vi "Graph ERD Read List.vi"(0 "GEA2 Reference In":refnum<k24>, 5 "GEA Inputs":T10={"Source"=240, "Destination"=35} {"Destination" format="%.0x"; "Source" format="%.0x"}, 7 "ERD_Data_Bundled_In":T1, 9 "ERD Graph Cntrl":T11={"ERD 3"={"ERD #"=0, "Data Type"=enum."uint16_t", "Scaler"=1}, "ERD 2"={"ERD #"=0, "Data Type"=enum."uint16_t", "Scaler"=1}, "ERD 1"={"ERD #"=0, "Data Type"=enum."uint16_t", "Scaler"=1}} {"ERD 1"."Scaler" min=1; "ERD 1"."ERD #" format="%.0x"; "ERD 2"."Scaler" min=1; "ERD 2"."ERD #" format="%.0x"; "ERD 3"."Scaler" min=1; "ERD 3"."ERD #" format="%.0x"}, 11 "Error In":errorcluster) -> (4 "GEA2 Reference Out":refnum<k24>, 6 "ERD Graph  Ind":T9, 8 "ERD_Data_Bundled_Out":T1, 15 "Error Out":errorcluster)   [LabVIEW 2014]
uses:
  Common/LabVIEW GEA2 Toolkit/LabVIEW_GEA2_Toolkit.lvlibp/type defs/ERD Read Data In.ctl
  Common/LabVIEW GEA2 Toolkit/LabVIEW_GEA2_Toolkit.lvlibp
  Common/LabVIEW GEA2 Toolkit/LabVIEW_GEA2_Toolkit.lvlibp/type defs/Data Type.ctl
  type defs/ERD_Graph.ctl
  type defs/ERD_Graph_All.ctl
  C:/Automation/DLLs/PC Dot Net/GeaCommunication.dll
  Common/LabVIEW GEA2 Toolkit/LabVIEW_GEA2_Toolkit.lvlibp/type defs/Source_Destination.ctl
  type defs/ATC_Data.ctl
  type defs/Redundant.ctl
  type defs/Version.ctl
  type defs/Algorithms.ctl
  type defs/ERD_Always_Show.ctl
  type defs/ERD_Data_Bundled.ctl
  type defs/Fault_Table_Info.ctl
  type defs/Cycle_Diag.ctl
panel:
  # "Wet Load Size"
  # "Dry Load Size"
  # "OOB"
  # "Software Version"
  # "Critical Version"
  # "Non-Critical"
  # "XML Crit Ver"
  # "XML Non-Crit"
  # "Daily Build"
  # "Wet Load Size"
  # "Dry Load Size"
  # "OOB"
  # "Software Version"
  # "Critical Version"
  # "Non-Critical"
  # "XML Crit Ver"
  # "XML Non-Crit"
  # "Daily Build"
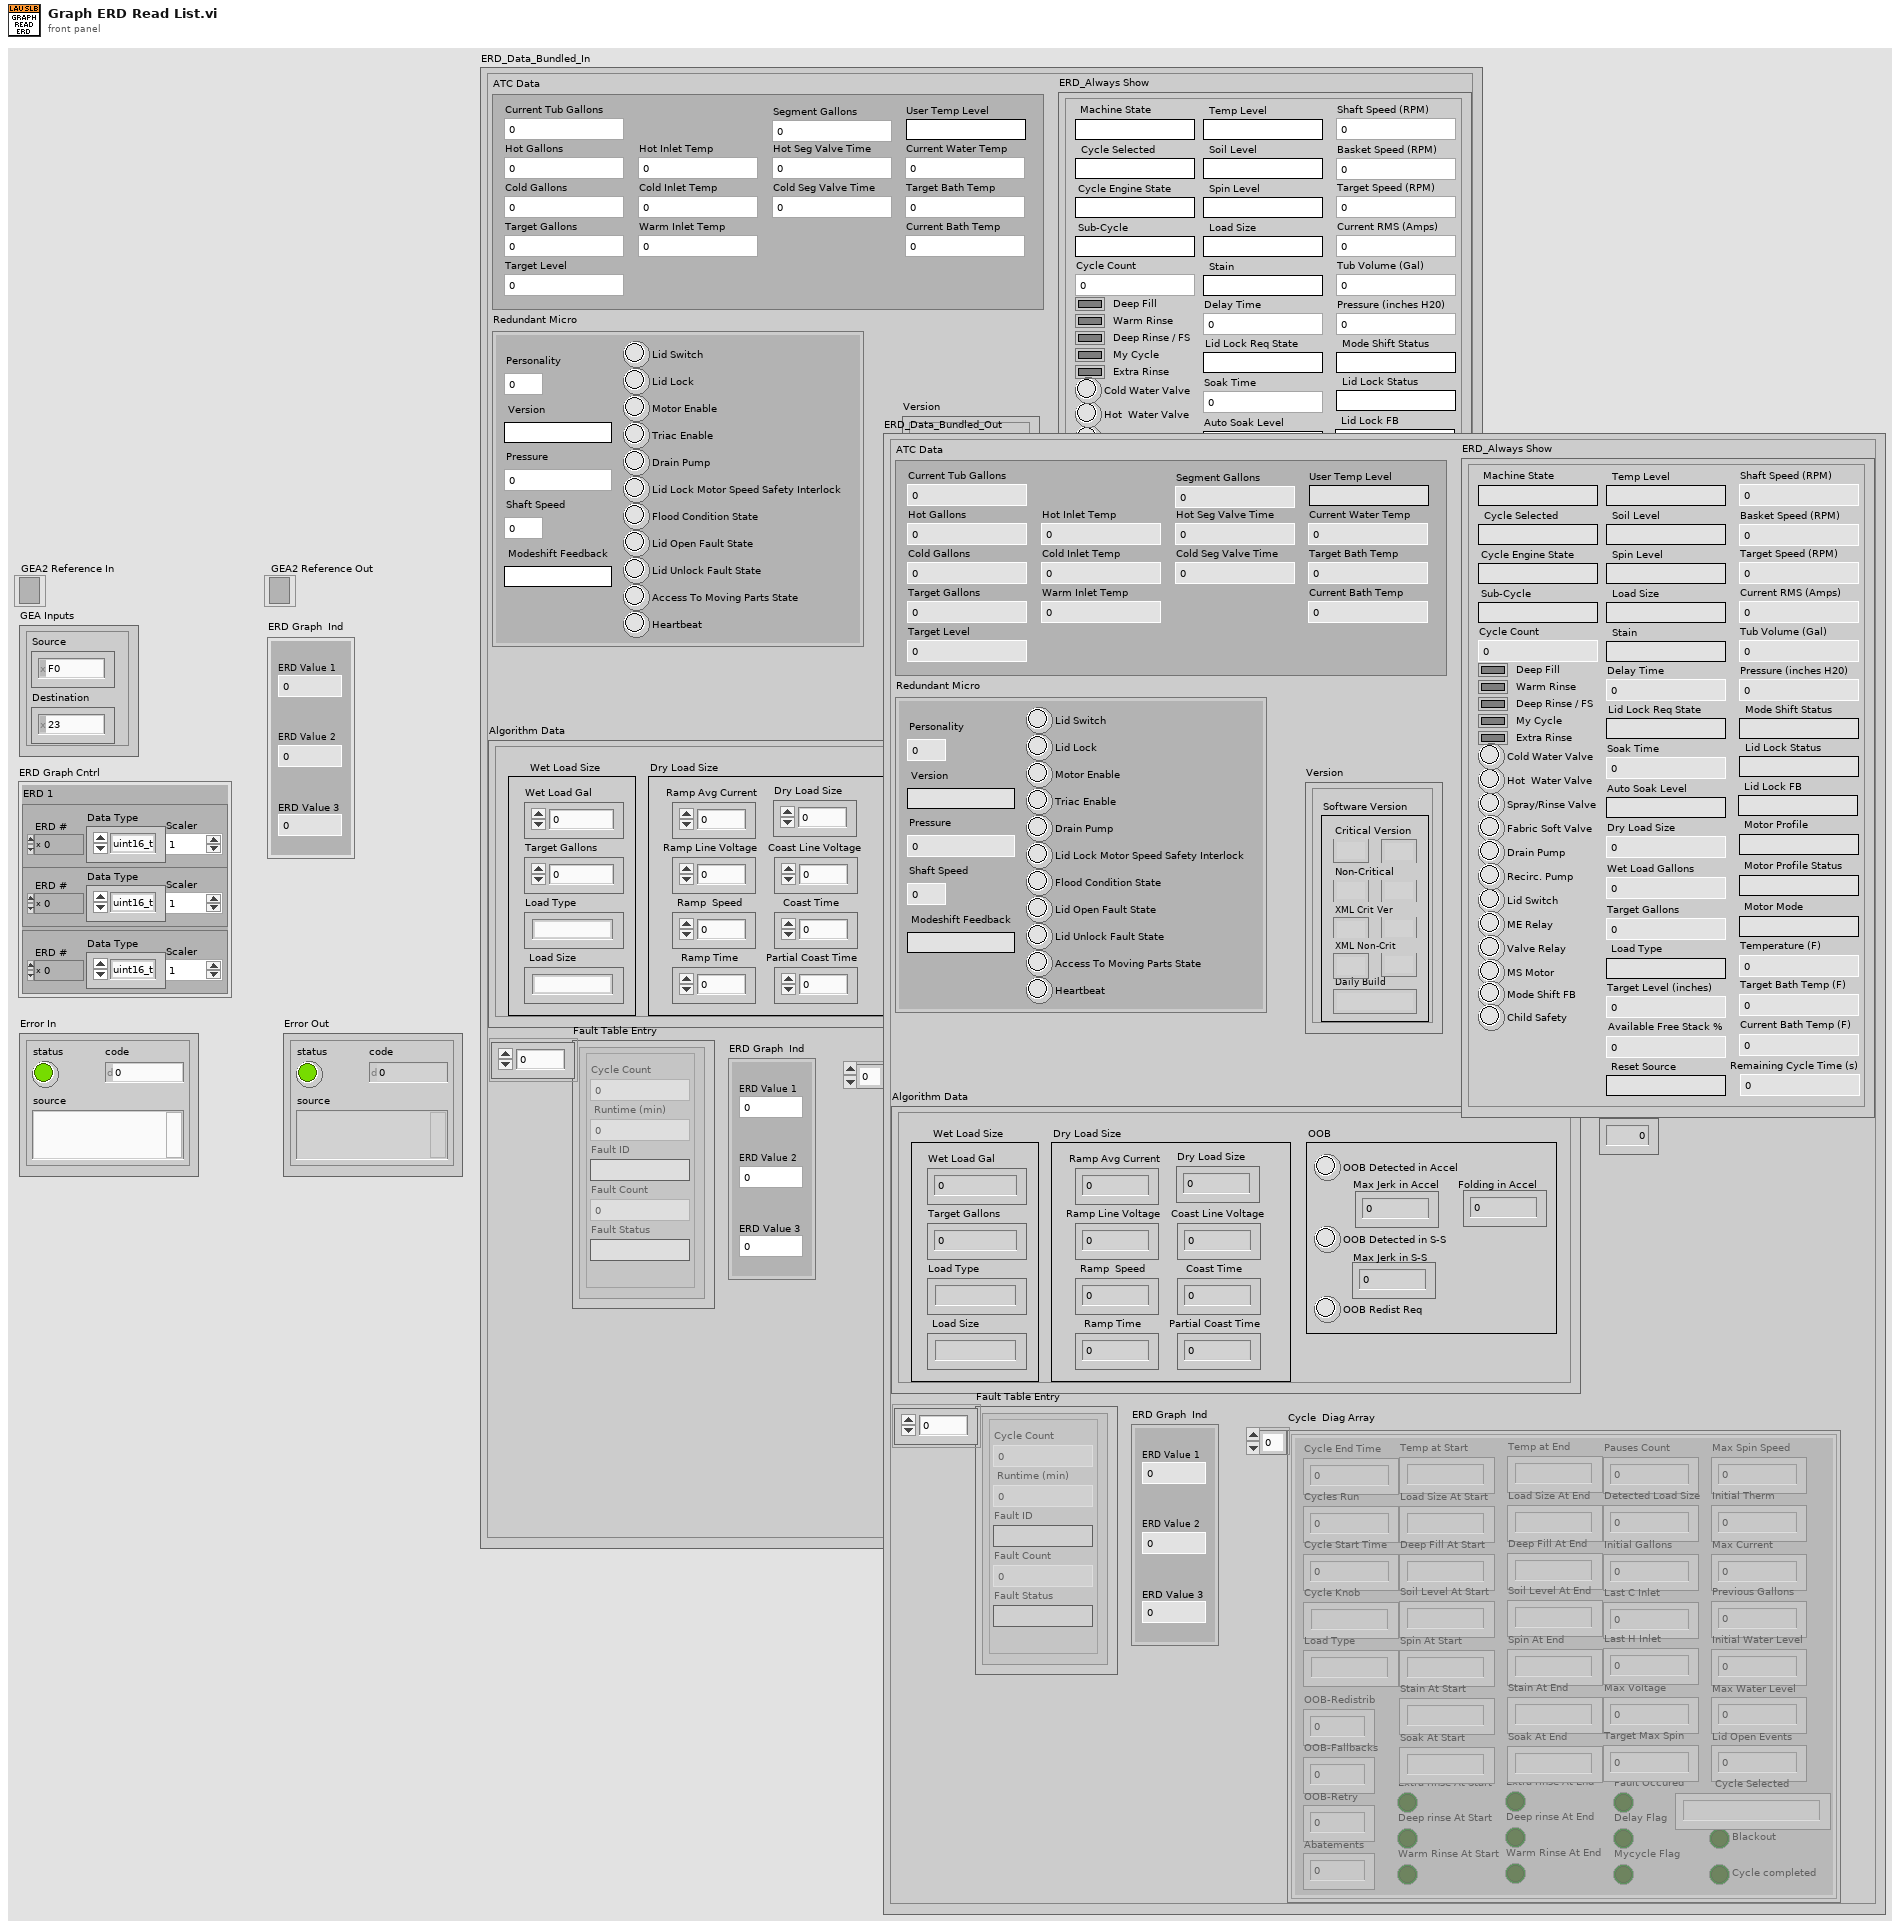
[diagram p1: front panel]
types:
  T1 = typedef "ERD_Data_Bundled.ctl" = cluster{"ATC Data":T2, "Redundant Micro":T3, "Version":T4, "Algorithm Data":T5, "ERD_Always Show":T6, "ERD Graph  Ind":cluster{"ERD Value 1":dbl, "ERD Value 2":dbl, "ERD Value 3":dbl}, "Personality Set":u8, "Fault Table Entry":T7[], "Cycle  Diag Array":T8[]}
  T2 = typedef "ATC_Data.ctl" = cluster{"Current Tub Gallons":dbl, "Hot Gallons":dbl, "Cold Gallons":dbl, "Target Gallons":dbl, "Current Water Temp":dbl, "Target Level":u32, "Target Bath Temp":dbl, "Current Bath Temp ":dbl, "Cold Inlet Temp":dbl, "Hot Inlet Temp":dbl, "Warm Inlet Temp":dbl, "Hot Seg Valve Time":u16, "Cold Seg Valve Time ":u16, "User Temp Level":string, "Segment Gallons":dbl}
  T3 = typedef "Redundant.ctl" = cluster{"Version":string, "Personality":u8, "Pressure ":dbl, "Shaft Speed":u16, "Modeshift Feedback":string, "Lid Switch":bool, "Lid Lock":bool, "Triac Enable":bool, "Drain Pump":bool, "Lid Lock Motor Speed Safety Interlock":bool, "Flood Condition State":bool, "Lid Open Fault State":bool, "Access To Moving Parts State":bool, "Heartbeat":bool, "Motor Enable":bool, "Lid Unlock Fault State":bool}
  T4 = typedef "Version.ctl" = cluster{"Critical Major":string, "Critical Minor":string, "Non-Critical Minor":string, "Non-Critical Major":string, "XML Crit Minor":string, "XMLCrit Major":string, "Daily Rev":string, "XML Non-crit Minor":string, "Xml Non-crit Major":string}
  T5 = typedef "Algorithms.ctl" = cluster{"Wet Load Gal":dbl, "Target Gallons":dbl, "Load Type":string, "Load Size":string, "Coast Time":u16, "Ramp Time":u16, "Ramp  Speed":u16, "Ramp Avg Current":dbl, "OOB Redist Req":bool, "OOB Detected in S-S":bool, "Folding in Accel":i32, "Max Jerk in Accel":i32, "Max Jerk in S-S":i32, "OOB Detected in Accel":bool, "Partial Coast Time":u16, "Dry Load Size":dbl, "Ramp Line Voltage ":dbl, "Coast Line Voltage":dbl}
  T6 = typedef "ERD_Always_Show.ctl" = cluster{"Basket Speed (RPM)":u16, "Machine State":string, "Tub Volume (Gal)":dbl, "Pressure (inches H20)":dbl, "Lid Switch ":bool, "Current RMS (Amps)":dbl, "Cycle Selected":string, "Lid Lock Status":string, "Mode Shift Status":string, "Spray/Rinse Valve":bool, "Fabric Soft Valve":bool, "Drain Pump":bool, "Recirc. Pump":bool, "Cycle Engine State":string, "Hot  Water Valve":bool, "Cold Water Valve":bool, "Motor Profile":string, "Motor Profile Status":string, "Motor Mode":string, "ME Relay":bool, "Cycle Count":u32, "Deep Rinse / FS":bool, "My Cycle":bool, "Soil Level":string, "Spin Level":string, "Stain":string, "Temp Level":string, "Load Size":string, "Delay Time":u16, "Soak Time":u16, "Deep Fill":bool, "Warm Rinse":bool, "Auto Soak Level":string, "Extra Rinse":bool, "Wet Load Gallons":dbl, "Target Gallons":dbl, "Sub-Cycle":string, "Load Type":string, "Target Level (inches)":u32, "Valve Relay":bool, "Dry Load Size":dbl, "Shaft Speed (RPM) ":u16, "MS Motor":bool, "Mode Shift FB":bool, "Target Bath Temp (F)":dbl, "Temperature (F)":dbl, "Current Bath Temp (F)":dbl, "Lid Lock FB":string, "Lid Lock Req State":string, "Remaining Cycle Time (s)":u32, "Available Free Stack %":u8, "Child Safety":bool, "Target Speed (RPM)":u16, "Reset Source":string}
  T7 = typedef "Fault_Table_Info.ctl" = cluster{"Cycle Count":u32, " Runtime (min) ":u32, "Fault Status":string, "Fault ID":string, "Fault Count":u16}
  T8 = typedef "Cycle_Diag.ctl" = cluster{"Cycle End Time":u32, "Cycles Run":u32, "Cycle Start Time":u32, "Cycle Knob":string, "Load Type":string, "OOB-Redistrib":u8, "OOB-Fallbacks":u8, "OOB-Retry":u8, "Temp at Start":string, "Load Size At Start":string, "Deep Fill At Start":string, "Soil Level At Start":string, "Spin At Start":string, "Extra rinse At Start":bool, "Deep rinse At Start":bool, "Stain At Start":string, "Soak At Start":string, "Warm Rinse At Start":bool, "Temp at End":string, "Load Size At End":string, "Deep Fill At End":string, "Soil Level At End":string, "Spin At End":string, "Extra rinse At End":bool, "Deep rinse At End":bool, "Stain At End":string, "Soak At End":string, "Warm Rinse At End":bool, "Pauses Count":u8, "Fault Occured":bool, "Delay Flag":bool, "Mycycle Flag":bool, "Blackout":bool, "Cycle completed":bool, "Detected Load Size":dbl, "Initial Gallons":dbl, "Last C Inlet ":dbl, "Max Voltage":dbl, "Target Max Spin":u16, "Max Spin Speed":u16, "Initial Therm":dbl, "Max Current":dbl, "Previous Gallons":dbl, "Initial Water Level":dbl, "Max Water Level":dbl, "Abatements ":u8, "Lid Open Events":u8, "Cycle Selected":string, "Last H Inlet ":dbl}
  T9 = cluster{"ERD Value 1":dbl, "ERD Value 2":dbl, "ERD Value 3":dbl}
  T10 = typedef "LabVIEW_GEA2_Toolkit.lvlibp/Source_Destination.ctl" = cluster{"Source":u8, "Destination":u8}
  T11 = typedef "ERD_Graph_All.ctl" = cluster{"ERD 3":T12, "ERD 2":T12, "ERD 1":T12}
  T12 = typedef "ERD_Graph.ctl" = cluster{"ERD #":u16, "Data Type":T13, "Scaler":u32}
  T13 = typedef "LabVIEW_GEA2_Toolkit.lvlibp/Data Type.ctl" = enum16{"string", "boolean", "uint8_t", "uint16_t", "uint32_t", "uint64_t", "int8_t", "int16_t", "int32_t", "int64_t"}
  T14 = typedef "LabVIEW_GEA2_Toolkit.lvlibp/ERD Read Data In.ctl" = cluster{"ERD Number":u16, "Data Type":T13}
  T15 = typedef "LabVIEW_GEA2_Toolkit.lvlibp/ERD Read Data Out.ctl" = cluster{"ERD Number":u16, "Data":string}
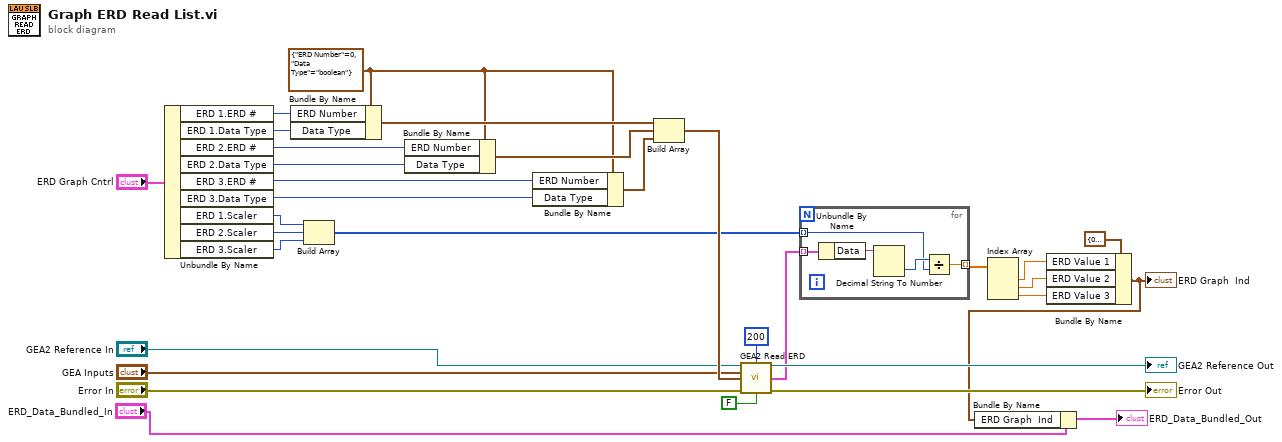
[diagram p0: block diagram]
diagram:
  w28 = T14 {"ERD Number"=0, "Data Type"=enum."boolean"} ("ERD Read Data In 2")
  n1 = Unbundle By Name("ERD Graph Cntrl") -> ("ERD 1.ERD #"=w22:u16, "ERD 1.Data Type"=w23:T13, "ERD 2.ERD #"=w24:u16, "ERD 2.Data Type"=w25:T13, "ERD 3.ERD #"=w26:u16, "ERD 3.Data Type"=w27:T13, "ERD 1.Scaler"=w15:u32, "ERD 2.Scaler"=w14:u32, "ERD 3.Scaler"=w13:u32)
  n2 = Bundle By Name(cluster=w28, "ERD Number"=w22, "Data Type"=w23) -> (w29:T14)
  n3 = Build Array(w15, w14, w13) -> (w12:u32[])
  n4 = Bundle By Name(cluster=w28, "ERD Number"=w24, "Data Type"=w25) -> (w30:T14)
  n5 = Bundle By Name(cluster=w28, "ERD Number"=w26, "Data Type"=w27) -> (w31:T14)
  n6 = Build Array(w29, w30, w31) -> (w21:T14[])
  n7 = call "GEA2 Read ERD.vi"("GEA2 Reference In"="GEA2 Reference In", "Read Timeout (ms)"=u32 200, "GEA Inputs"="GEA Inputs", "Read ERD List"=w21, "Error In"="Error In", "Verify ERD Response?"=FALSE) -> ("GEA2 Reference Out"=→"GEA2 Reference Out":refnum<k24>, "ERD Data Out"=w11:T15[], "Error Out"=→"Error Out":errorcluster)  [unwired: 6 in, 1 out]
  n8 = for {
    tunnel: w12 -> [w34] mode=indexing
    tunnel: w11 -> [w37] mode=indexing
    tunnel: [w33] -> w10 mode=indexing
    n9 = Unbundle By Name(w37) -> ("Data"=w36:string)
    n10 = Decimal String To Number(string=w36) -> (number=w35:i32)  [unwired: 2 in, 1 out]
    n11 = Divide(x=w35, y=w34) -> (x/y=w33:dbl)
  }
  n12 = Index Array(array=w10) -> (element #1=w8:dbl, element #2=w7:dbl, element #3=w6:dbl)  [unwired: 3 in]
  n13 = Bundle By Name(cluster=T9 {"ERD Value 1"=0.0, "ERD Value 2"=0.0, "ERD Value 3"=0.0} ("ERD Graph  Ind"), "ERD Value 1"=w8, "ERD Value 2"=w7, "ERD Value 3"=w6) -> (w2:T9)
  "ERD Graph  Ind" <- w2
  n14 = Bundle By Name(cluster="ERD_Data_Bundled_In", "ERD Graph  Ind"=w2) -> (→"ERD_Data_Bundled_Out":T1)
